vi "FindVIEWs.vi"(8 "error in (no error)":errorcluster, 11 "VIEW in":refnum<class "VIEW.lvclass">) -> (0 "error out":errorcluster, 3 "VIEW out":refnum<class "VIEW.lvclass">)   [LabVIEW 2013, in "VIEW.lvclass"]
uses:
  VIEW.lvclass
  VIEW.lvclass/VIEW.ctl
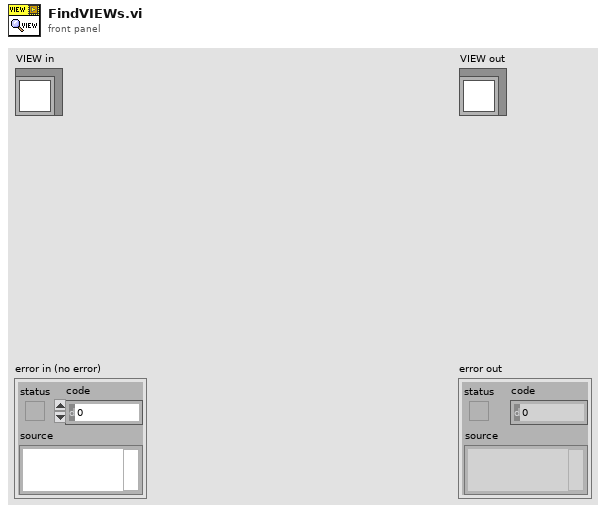
[diagram p1: front panel]
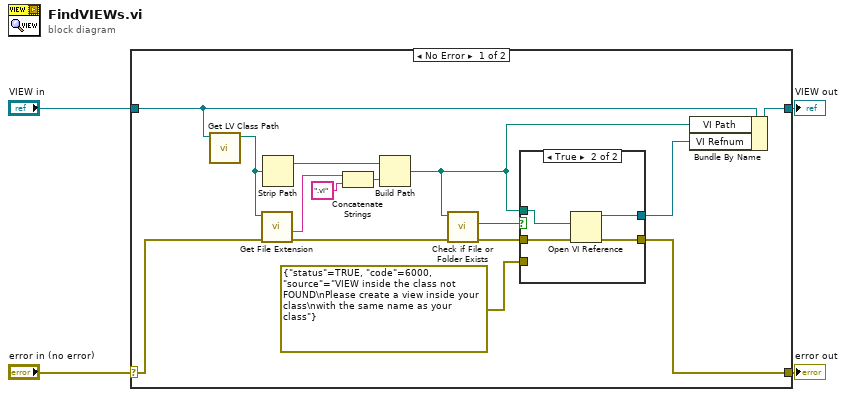
[diagram p0: block diagram]
diagram:
  n1 = case shown="No Error" "error in (no error)" {
    selector: "error in (no error)" -> [w12 w26]
    tunnel: [w13 w26] -> w3
    tunnel: [w15 w25] -> w1
    tunnel: "VIEW in" -> [w10 w25]
    frame No Error {
      n2 = call <vilib>:"Get LV Class Path.vi"("object"=w10) -> ("class path"=w9:path)  [unwired: 9 in, 1 out]
      n3 = call <vilib>:"Get File Extension.vi"("error in (no error)"=w12, "file"=w9) -> ("error out"=w11:errorcluster, "filename without extension"=w19:string)  [unwired: 6 in, 2 out]
      n4 = Strip Path(path=w9) -> (stripped path=w16:path)  [unwired: 1 out]
      n5 = Concatenate Strings(w19, ".vi" ("string")) -> (w17:string)
      n6 = Build Path(base path=w16, name or relative path=w17) -> (appended path=w7:path)
      n7 = call <vilib>:"Check if File or Folder Exists.vi"("error in (no error)"=w11, "path"=w7) -> ("error out"=w8:errorcluster, "file or folder exists?"=w6:bool)  [unwired: 7 in, 1 out]
      n8 = case shown="True" w6 {
        tunnel: [_ w24] -> w14
        tunnel: [w20 w23] -> w13
        tunnel: w8 -> [_ w22]
        tunnel: w7 -> [_ w21]
        tunnel: errorcluster {"status"=TRUE, "code"=6000, "source"="VIEW inside the class not FOUND\nPlease create a view inside your class\nwith the same name as your class"} ("error out") -> [w20 _]
        frame False {
        }
        frame True {
          n9 = Open VI Reference(vi path=w21, error in (no error)=w22) -> (vi reference=w24:refnum<vi>, error out=w23:errorcluster)  [unwired: 4 in]
        }
      }
      n10 = Bundle By Name(cluster=w10, "VI Path"=w7, "VI Refnum"=w14) -> (w15:refnum<class "VIEW.lvclass">)
    }
    frame Error {
    }
  }
  "error out" <- w3
  "VIEW out" <- w1
